vi "ziPollData.vi"(8 "Error In":errorcluster, 9 "Data In":T1, 10 "TimeOut ms (50)":i32=50, 11 "Handle In":T3 {"Handle" format="0x%08x"; "Conn" format="0x%08x"}) -> (0 "Error Out":errorcluster, 1 "Data Out":T1, 2 "PathArray":string[](array[string]), 3 "Handle Out":T3 {"Handle" format="0x%08x"; "Conn" format="0x%08x"}, 5 "Timed Out":bool, 7 "ziDataType":T4)   [LabVIEW 2018, in "Zurich Instruments LabOne.lvlib"]
doc: "---Obsolete---\n(Please use ziPollDataEx instead)\nThis vi is <b>obsolete</b>. Use ziPollDataEx.vi in combination with ziGetEvent.vi instead.\n\nThis vi returns immediately if data is pending. Otherwise it waits for data for up to <b>TimeOut</b> milliseconds. All value changes that occur in nodes that have been subscribed to or in children of nodes that have been subscribed to, are sent from the Data Server to the ziAPI session. When no event was available within <b>TimeOut</b> milliseconds, the ziValueType field will be ZI_DATA_NONE and <b>Timed Out</b> will be true. Otherwise these fields hold the values corresponding to the event occurred."
uses:
  Zurich Instruments LabOne.lvlib
  <instrlib>/Zurich Instruments LabOne/Private/ziLV64.framework
  ziGetEventAuxInSample.vi
  ziGetEventDIOSample.vi
  ziGetEventScopeWave.vi
  ziGetEventByteArray.vi
  ziGetEventTreeChange.vi
  ziTypeDemodSample.ctl
  ziTypeHandle.ctl
  ziTypePollData.ctl
  ziTypePollType.ctl
panel:
  # "Obsolete (2013-11)\nUse ziPollDataEx instead"
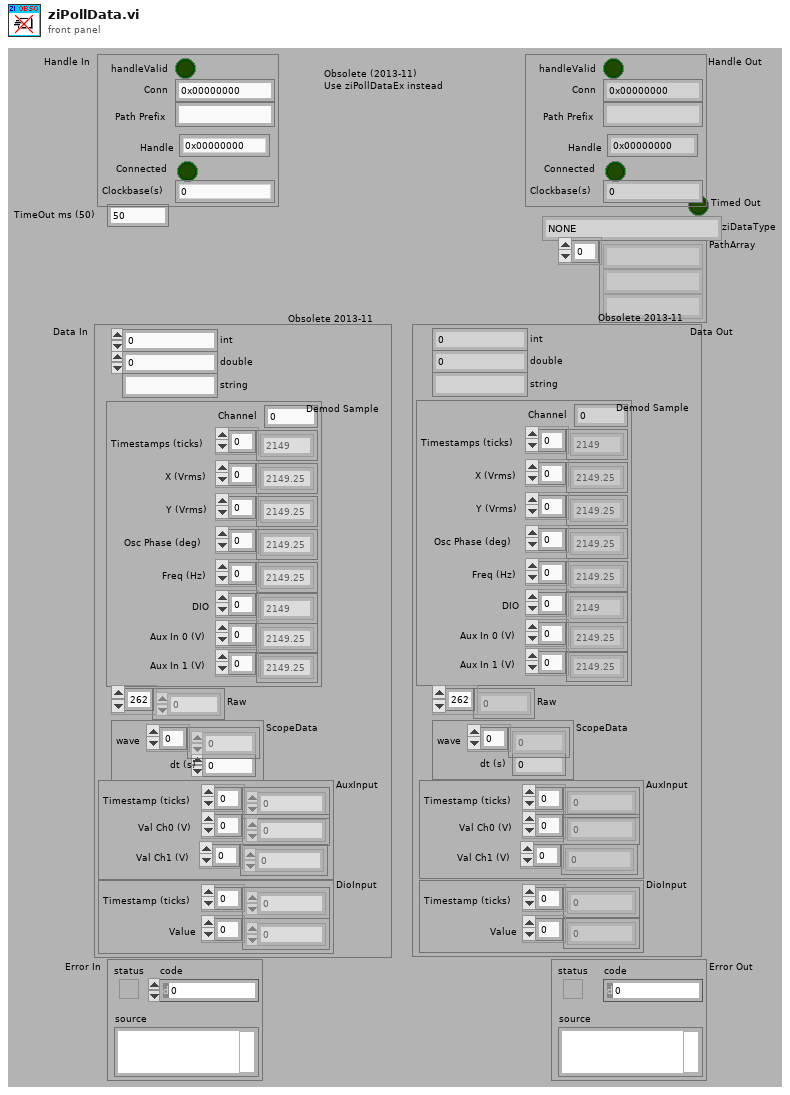
[diagram p1: front panel]
types:
  T1 = typedef "Zurich Instruments LabOne.lvlib/ziTypePollData.ctl" = cluster{"double":dbl, "Demod Sample":T2, "string":string, "Raw":u8[], "int":i32, "ScopeData":cluster{"wave":i16[], "dt (s)":dbl}, "DioInput":cluster{"Timestamp (ticks)":u64[], "Value":u32[]}, "AuxInput":cluster{"Timestamp (ticks)":u64[], "Val Ch0 (V)":dbl[], "Val Ch1 (V)":dbl[]}}
  T2 = typedef "Zurich Instruments LabOne.lvlib/ziTypeDemodSample.ctl" = cluster{"Channel":i32, "Timestamps (ticks)":u64[], "X (Vrms)":dbl[], "Y (Vrms)":dbl[], "Osc Phase (deg)":dbl[], "Freq (Hz)":dbl[], "DIO":u32[], "Aux In 0 (V)":dbl[], "Aux In 1 (V)":dbl[]}
  T3 = typedef "Zurich Instruments LabOne.lvlib/ziTypeHandle.ctl" = cluster{"handleValid":bool, "Conn":u64, "Path Prefix":string, "Handle":u64, "Connected":bool, "Clockbase(s)":dbl}
  T4 = typedef "Zurich Instruments LabOne.lvlib/ziTypePollType.ctl" = enum16{"NONE", "DOUBLE_DATA", "INTEGER_DATA", "DEMOD_SAMPLE", "SCOPE_WAVE_HF2", "AUXIN_SAMPLE", "DIO_SAMPLE", "BYTE_ARRAY", "PWA_WAVE", "9", "10", "11", "12", "13", "14", "15", "TREE_CHANGE_DEPRI", "17", "ERROR", "19", "20", "21", "22", "23", "24", "25", "26", "27", "28", "29", "30", "31", "DOUBLE_DATA_TS", "INTEGER_DATA_TS", "34", "SCOPE_WAVE", "SCOPE_WAVE_EX", "37", "BYTE_ARRAY_TS", "39", "40", "41", "42", "43", "44", "45", "CNT_DATA", "47", "TREE_CHANGE", "49", "50", "51", "52", "53", "54", "55", "56", "57", "58", "59", "60", "61", "62", "63", "SWEEPER_DATA", "SPECTRUM_DATA", "ADVISOR_DATA", "VECTOR_DATA", "IMP_DATA"}
  T5 = typedef "Zurich Instruments LabOne.lvlib/ziTypeScopeWave.ctl" = cluster{"Timestamp (ticks)":u64, "Timestamp Trigger (ticks)":u64, "dt (s)":dbl, "Channel Enable":u8[], "Channel Input":enum8{"Signal Input 1", "Signal Input 2", "Trigger Input 1", "Trigger Input 2", "Aux Output 1", "Aux Output 2", "Aux Output 3", "Aux Output 4", "Aux Input 1", "Aux Input 2"}[], "Trigger Enable":u64, "Trigger Input":u64, "Channel BW Limit":u8[], "Channel Math":u8[], "Channel Scaling":sgl[], "Sequence Number":u32, "Segment Number":u32, "Block Number":u32, "Data Transfer Mode":enum8{"Single Transfer", "Block Transfer", "Continuous Transfer", "FFT Single Transfer"}, "Block Marker":enum8{"None", "End of Block"}, "Flags":u8, "Sample Format":enum8{"Int16", "Int32", "Float32", "reserved", "Int16 Interleaved", "Int32 Interleaved", "Float32 Interleaved"}, "Sample Count":u32, "Channel Offset":dbl[], "Data Int16":i16[], "Data Int32":i32[], "Data Float":sgl[], "Total Samples":u64}
  T6 = cluster{"Timestamp (ticks)":u64[], "Val Ch0 (V)":dbl[], "Val Ch1 (V)":dbl[]}
  T7 = typedef "Zurich Instruments LabOne.lvlib/ziTypeAuxInSample.ctl" = cluster{"Timestamp (ticks)":u64[], "Val Ch0 (V)":dbl[], "Val Ch1 (V)":dbl[]}
  T8 = cluster{"Timestamp (ticks)":u64[], "Value":u32[]}
  T9 = typedef "Zurich Instruments LabOne.lvlib/ziTypeByteArray.ctl" = cluster{"Timestamp (ticks)":u64[], "string":string[]}
  T10 = typedef "Zurich Instruments LabOne.lvlib/ziTypeTreeChange.ctl" = cluster{"Timestamp (ticks)":u64, "Action":enum32{"Remove", "Add", "Change"}, "Name":string}
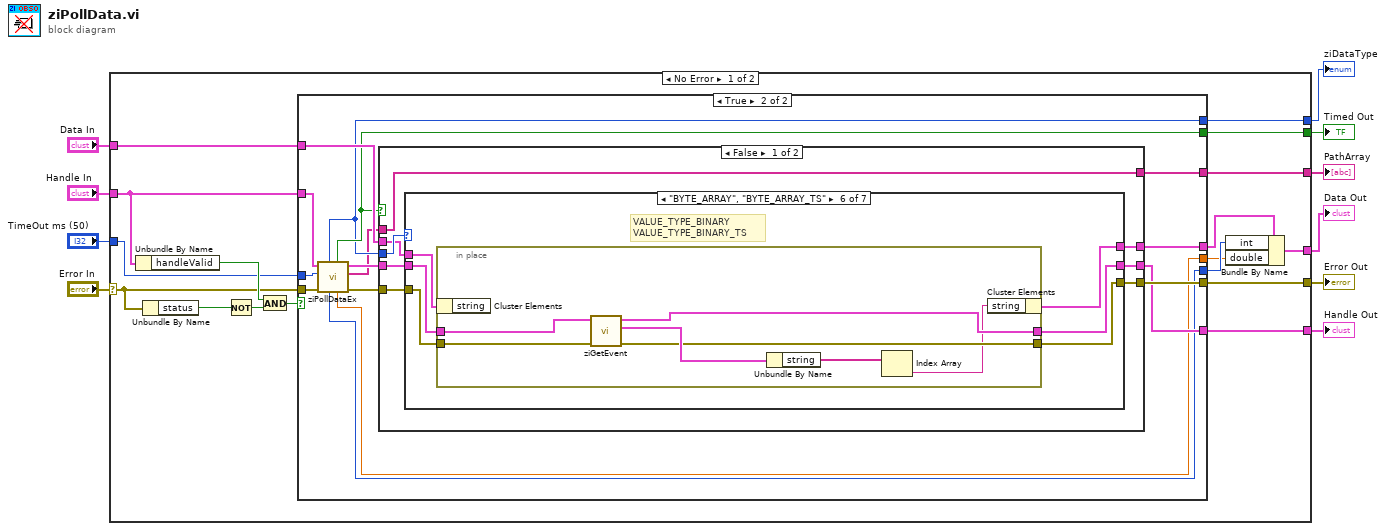
[diagram p0: block diagram]
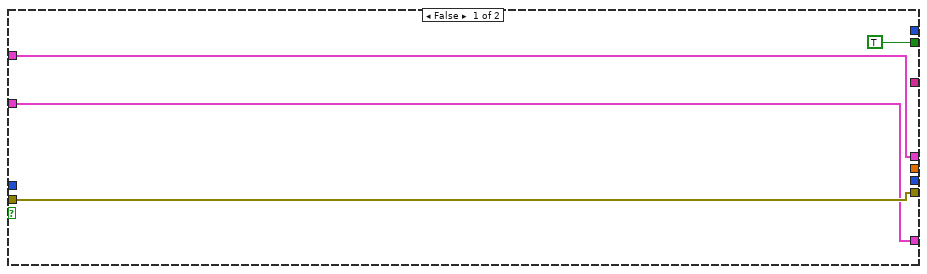
[diagram p2: hidden frame]
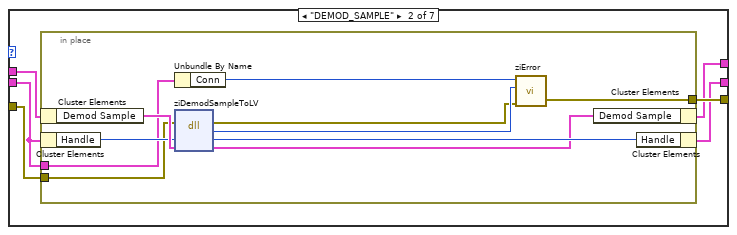
[diagram p4: hidden frame]
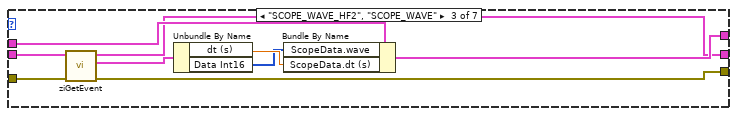
[diagram p5: hidden frame]
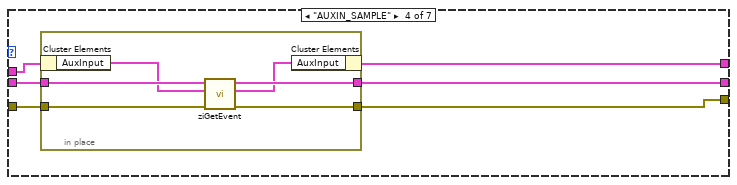
[diagram p6: hidden frame]
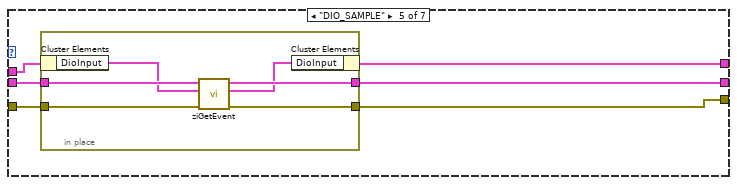
[diagram p7: hidden frame]
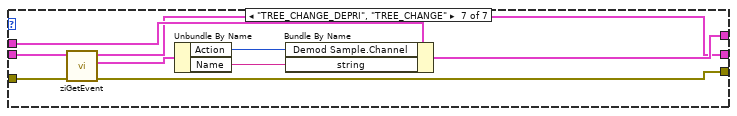
[diagram p8: hidden frame]
diagram:
  n1 = case shown="No Error" "Error In" {
    selector: "Error In" -> [w11 w133]
    tunnel: [w27 w133] -> w10
    tunnel: [w26 _] -> w9
    tunnel: [w24 w134] -> w8
    tunnel: "Data In" -> [w23 w134]
    tunnel: [w22 _] -> w6
    tunnel: [w17 w135] -> w5
    tunnel: [w16 w132] -> w4
    tunnel: "Handle In" -> [w13 w135]
    tunnel: "TimeOut ms (50)" -> [w12 w132]
    frame No Error {
      n2 = Unbundle By Name(w13) -> ("handleValid"=w20:bool)
      n3 = Unbundle By Name(w11) -> ("status"=w19:bool)
      n4 = Not(x=w19) -> (.not. x?=w18:bool)
      n5 = And(x=w20, y=w18) -> (x .and. y?=w21:bool)
      n6 = case shown="True" w21 {
        tunnel: w11 -> [w31 w37]
        tunnel: [w31 w46] -> w27
        tunnel: [_ w45] -> w26
        tunnel: [TRUE w40] -> w22
        tunnel: w23 -> [w29 w44]
        tunnel: [w29 w43] -> w25
        tunnel: w13 -> [w28 w41]
        tunnel: [w28 w42] -> w17
        tunnel: [_ w33] -> w16
        tunnel: [_ w34] -> w15
        tunnel: [_ w36] -> w14
        tunnel: w12 -> [_ w35]
        frame False {
        }
        frame True {
          n7 = call "ziPollDataEx.vi"("error in"=w37, "Timeout ms (50)"=w35, "Handle In"=w41) -> ("error out"=w38:errorcluster, "PathArray"=w32:string[], "Handle Out"=w39:T3, "Value Double"=w36:dbl, "Timed Out"=w40:bool, "Value Int"=w34:i32, "ziValueType"=w33:T4)  [unwired: 1 in, 1 out]
          n8 = case shown="False" w40 {
            tunnel: w33 -> [w54 _]
            tunnel: w38 -> [w53 w131]
            tunnel: [w52 w131] -> w46
            tunnel: [w47 _] -> w45
            tunnel: w44 -> [w51 w130]
            tunnel: [w50 w130] -> w43
            tunnel: w39 -> [w49 w129]
            tunnel: [w48 w129] -> w42
            tunnel: w32 -> [w47 _]
            frame False {
              n9 = case shown="\"BYTE_ARRAY\", \"BYTE_ARRAY_TS\"" w54 {
                tunnel: w53 -> [w57 w63 w80 w87 w99 w112 w122]
                tunnel: [w57 w62 w76 w85 w97 w109 w120] -> w52
                tunnel: w51 -> [w56 w61 w82 w84 w96 w108 w128]
                tunnel: [w56 w60 w81 w83 w95 w107 w127] -> w50
                tunnel: w49 -> [w55 w58 w75 w88 w100 w111 w126]
                tunnel: [w55 w59 w74 w86 w98 w110 w121] -> w48
                frame Default {
                }
                frame "DEMOD_SAMPLE" {
                  n10 = in-place {
                    in-place-border: w63 -> [w69]
                    in-place-border: [w67] -> w62
                    in-place-border: w58 -> [w65]
                    n11 = in-place-cluster #1(w61) -> ("Demod Sample"=w73:T2)
                    n12 = in-place-cluster #2(w58) -> ("Handle"=w72:u64)
                    n13 = Unbundle By Name(w65) -> ("Conn"=w64:u64)
                    n14 = dll-call lib="Applications/National Instruments/LabVIEW 2019 64-bit/instr.lib/Zurich Instruments LabOne/Private/ziLV*.*" fn="ziDemodSampleToLV"(error in=w69, "ziEventBuffer"=w72, "DemodSample"=w73) -> (error out=w68:errorcluster, "return type"=w70:u32, "ziEventBuffer"=w71:u64, "DemodSample"=w66:T2)  [unwired: 2 in, 1 out]
                    n15 = call "ziError.vi"("Conn"=w64, "ziErrorCode"=w70, "Error In"=w68) -> ("Error Out"=w67:errorcluster)  [unwired: 2 in, 1 out]
                    n16 = in-place-cluster #1("Demod Sample"=w66) -> (w60:T1)
                    n17 = in-place-cluster #2("Handle"=w71) -> (w59:T3)
                  }
                }
                frame "SCOPE_WAVE_HF2", "SCOPE_WAVE" {
                  n18 = call-poly "ziGetEvent.vi"("Error In"=w80, "Handle In"=w75) -> ("Error Out"=w76:errorcluster, "ScopeWave Out"=w79:T5, "Handle Out"=w74:T3)  [unwired: 7 in]
                  n19 = Unbundle By Name(w79) -> ("dt (s)"=w78:dbl, "Data Int16"=w77:i16[])
                  n20 = Bundle By Name(cluster=w82, "ScopeData.wave"=w77, "ScopeData.dt (s)"=w78) -> (w81:T1)
                }
                frame "AUXIN_SAMPLE" {
                  n21 = in-place {
                    in-place-border: w88 -> [w94]
                    in-place-border: w87 -> [w93]
                    in-place-border: [w92] -> w86
                    in-place-border: [w91] -> w85
                    n22 = in-place-cluster #3(w84) -> ("AuxInput"=w90:T6)
                    n23 = call-poly "ziGetEvent.vi"("Error In"=w93, "AuxIn In"=w90, "Handle In"=w94) -> ("Error Out"=w91:errorcluster, "AuxIn Out"=w89:T7, "Handle Out"=w92:T3)  [unwired: 6 in]
                    n24 = in-place-cluster #3("AuxInput"=w89) -> (w83:T1)
                  }
                }
                frame "DIO_SAMPLE" {
                  n25 = in-place {
                    in-place-border: w100 -> [w106]
                    in-place-border: w99 -> [w105]
                    in-place-border: [w104] -> w98
                    in-place-border: [w103] -> w97
                    n26 = in-place-cluster #4(w96) -> ("DioInput"=w102:T8)
                    n27 = call-poly "ziGetEvent.vi"("Error In"=w105, "DIOIn"=w102, "Handle In"=w106) -> ("Error Out"=w103:errorcluster, "DIO Out"=w101:T8, "Handle Out"=w104:T3)  [unwired: 6 in]
                    n28 = in-place-cluster #4("DioInput"=w101) -> (w95:T1)
                  }
                }
                frame "BYTE_ARRAY", "BYTE_ARRAY_TS" {
                  # "VALUE_TYPE_BINARY\nVALUE_TYPE_BINARY_TS"
                  n29 = in-place {
                    in-place-border: w112 -> [w119]
                    in-place-border: w111 -> [w118]
                    in-place-border: [w117] -> w110
                    in-place-border: [w115] -> w109
                    n30 = in-place-cluster #5(w108) -> ()  [unwired: 1 out]
                    n31 = call-poly "ziGetEvent.vi"("Error In"=w119, "Handle In"=w118) -> ("Error Out"=w115:errorcluster, "ByteArray Out"=w116:T9, "Handle Out"=w117:T3)  [unwired: 7 in]
                    n32 = Unbundle By Name(w116) -> ("string"=w114:string[])
                    n33 = Index Array(array=w114) -> (element=w113:string)  [unwired: 1 in]
                    n34 = in-place-cluster #5("string"=w113) -> (w107:T1)
                  }
                }
                frame "TREE_CHANGE_DEPRI", "TREE_CHANGE" {
                  n35 = call-poly "ziGetEvent.vi"("Error In"=w122, "Handle In"=w126) -> ("Error Out"=w120:errorcluster, "TreeChange Out"=w125:T10, "Handle Out"=w121:T3)  [unwired: 7 in]
                  n36 = Unbundle By Name(w125) -> ("Action"=w123:enum32{"Remove", "Add", "Change"}, "Name"=w124:string)
                  n37 = Bundle By Name(cluster=w128, "Demod Sample.Channel"=w123, "string"=w124) -> (w127:T1)
                }
              }
            }
            frame True {
            }
          }
        }
      }
      n38 = Bundle By Name(cluster=w25, "int"=w15, "double"=w14) -> (w24:T1)
    }
    frame Error {
    }
  }
  "Error Out" <- w10
  "ziDataType" <- w4
  "Timed Out" <- w6
  "Handle Out" <- w5
  "PathArray" <- w9
  "Data Out" <- w8
